vi "Plot IMU.vi"(8 "Target Lossy Data":T2) -> (3 "IMU Waveform":T1)   [LabVIEW 2018]
uses:
  Target Lossy Data.ctl
  Sensor Data.ctl
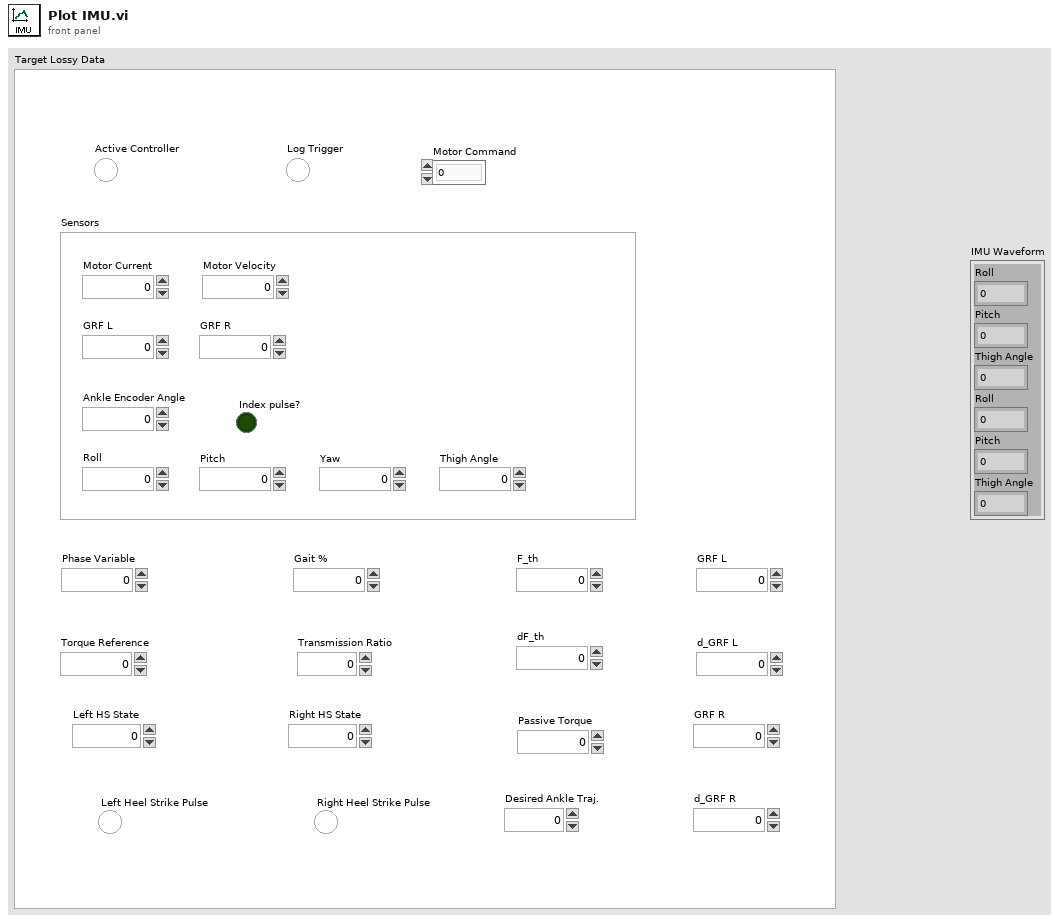
[diagram p1: front panel]
types:
  T1 = cluster{"Roll":dbl, "Pitch":dbl, "Thigh Angle":dbl, "Roll":dbl, "Pitch":dbl, "Thigh Angle":dbl}
  T2 = typedef "Target Lossy Data.ctl" = cluster{"Active Controller":bool, "Log Trigger":bool, "Sensors":T3, "Motor Command":dbl, "Phase Variable":dbl, "Left HS State":u32, "Left Heel Strike Pulse":bool, "Gait %":dbl, "Torque Reference":dbl, "Passive Torque":dbl, "F_th":dbl, "dF_th":dbl, "d_GRF L":dbl, "GRF L":dbl, "Transmission Ratio":dbl, "Desired Ankle Traj.":dbl, "Right HS State":u32, "Right Heel Strike Pulse":bool, "d_GRF R":dbl, "GRF R":dbl}
  T3 = typedef "Sensor Data.ctl" = cluster{"Motor Current":dbl, "Motor Velocity":dbl, "Ankle Encoder Angle":dbl, "GRF L":dbl, "GRF R":dbl, "Index pulse?":bool, "Roll":dbl, "Pitch":dbl, "Yaw":dbl, "Thigh Angle":dbl}
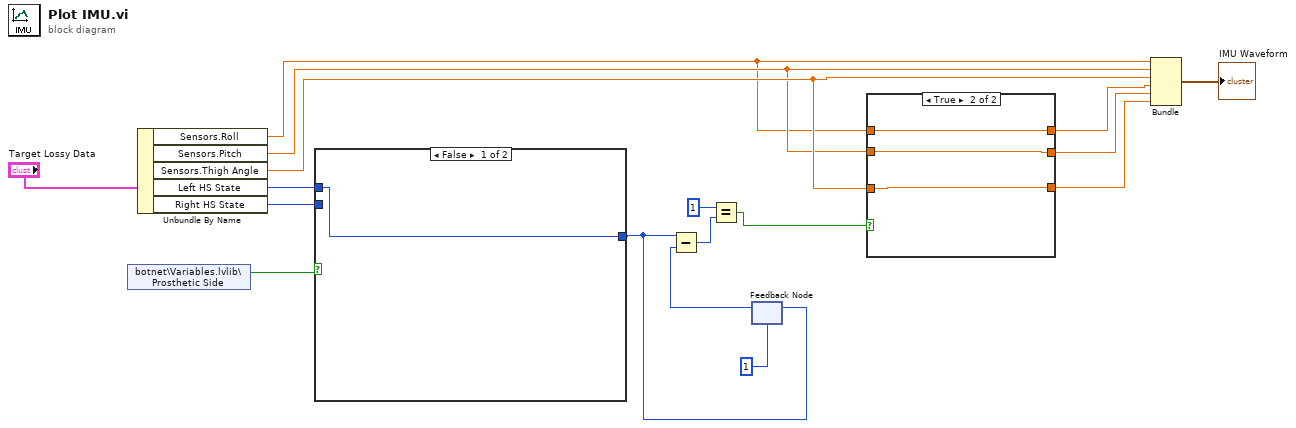
[diagram p0: block diagram]
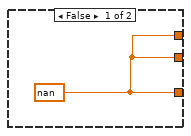
[diagram p2: hidden frame]
diagram:
  n1 = shared-variable "botnet\\Variables.lvlib\\Prosthetic Side"() -> (w16:bool)  [unwired: 1 in, 1 out]
  n2 = Unbundle By Name("Target Lossy Data") -> ("Sensors.Roll"=w4:dbl, "Sensors.Pitch"=w5:dbl, "Sensors.Thigh Angle"=w7:dbl, "Left HS State"=w14:u32, "Right HS State"=w15:u32)
  n3 = case shown="False" w16 {
    tunnel: w15 -> [_ w19]
    tunnel: w14 -> [w18 _]
    tunnel: [w18 w19] -> w9
    frame False {
    }
    frame True {
    }
  }
  n4 = feedback #1(1) -> (w12:u32)
  n5 = Subtract(x=w9, y=w12) -> (x-y=w10:u32)
  n6 = Equal?(x=1, y=w10) -> (x = y?=w8:bool)
  n7 = feedback-in #1(w9) -> ()
  n8 = case shown="True" w8 {
    tunnel: w7 -> [_ w23]
    tunnel: [w20 w23] -> w6
    tunnel: [w20 w22] -> w3
    tunnel: [w20 w21] -> w2
    tunnel: w5 -> [_ w22]
    tunnel: w4 -> [_ w21]
    frame False {
      w20 = nan
    }
    frame True {
    }
  }
  n9 = Bundle("Roll"=w4, "Pitch"=w5, "Thigh Angle"=w7, "Roll"=w2, "Pitch"=w3, "Thigh Angle"=w6) -> (→"IMU Waveform":T1)  [unwired: 1 in]
